vi "Load INI Config.vi"(8 "error in (no error)":errorcluster, 11 "Builder in":refnum<class "Builder.lvclass">) -> (0 "error out":errorcluster, 3 "Builder out":refnum<class "Builder.lvclass">)   [LabVIEW 2019, in "Builder.lvclass"]
uses:
  Builder.lvclass
  Builder.lvclass/Builder.ctl
  INI Parsing/PPL INI Parsing.lvlib
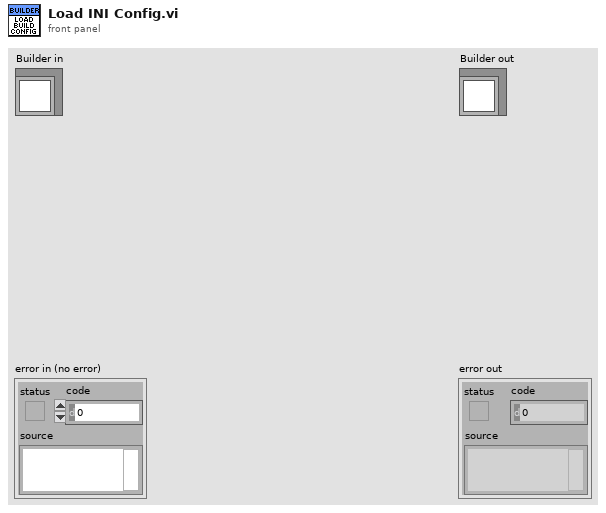
[diagram p1: front panel]
types:
  T1 = typedef "PPL INI Parsing.lvlib/Build Configuration.ctl" = cluster{"SV Pairs":string[][], "Description":string}
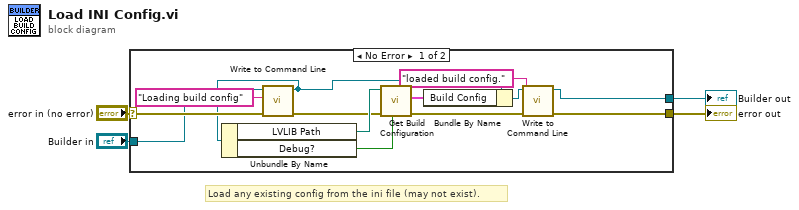
[diagram p0: block diagram]
diagram:
  # "Load any existing config from the ini file (may not exist)."
  n1 = case shown="No Error" "error in (no error)" {
    selector: "error in (no error)" -> [w16 w19]
    tunnel: [w8 w19] -> w3
    tunnel: [w6 w18] -> w1
    tunnel: "Builder in" -> [w11 w18]
    frame No Error {
      n2 = call "Write to Command Line.vi"("error in (no error)"=w16, "Message"="Loading build config", "Builder in"=w11) -> ("error out"=w12:errorcluster, "Builder out"=w10:refnum<class "Builder.lvclass">)  [unwired: 7 in]
      n3 = Unbundle By Name(w10) -> ("LVLIB Path"=w17:path, "Debug?"=w15:bool)
      n4 = call "Get Build Configuration.vi"("Debug Build?"=w15, "error in (no error)"=w12, "Library Path"=w17) -> ("error out"=w14:errorcluster, "Build Config"=w13:T1)  [unwired: 6 in, 1 out]
      n5 = Bundle By Name(cluster=w10, "Build Config"=w13) -> (w7:refnum<class "Builder.lvclass">)
      n6 = call "Write to Command Line.vi"("error in (no error)"=w14, "Message"="loaded build config.", "Builder in"=w7) -> ("error out"=w8:errorcluster, "Builder out"=w6:refnum<class "Builder.lvclass">)  [unwired: 7 in]
    }
    frame Error {
    }
  }
  "error out" <- w3
  "Builder out" <- w1
